vi "Shooter_Sucker_Feed_Mix.vi"(2 "Axis_Y":dbl, 3 "Axis_X":dbl) -> (0 "Suck_Feeder_Out":dbl, 1 "Shoot_Feeder_Out":dbl)   [LabVIEW 2011]
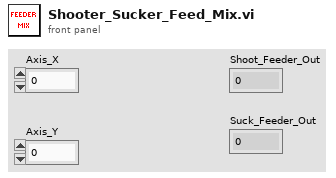
[diagram p1: front panel]
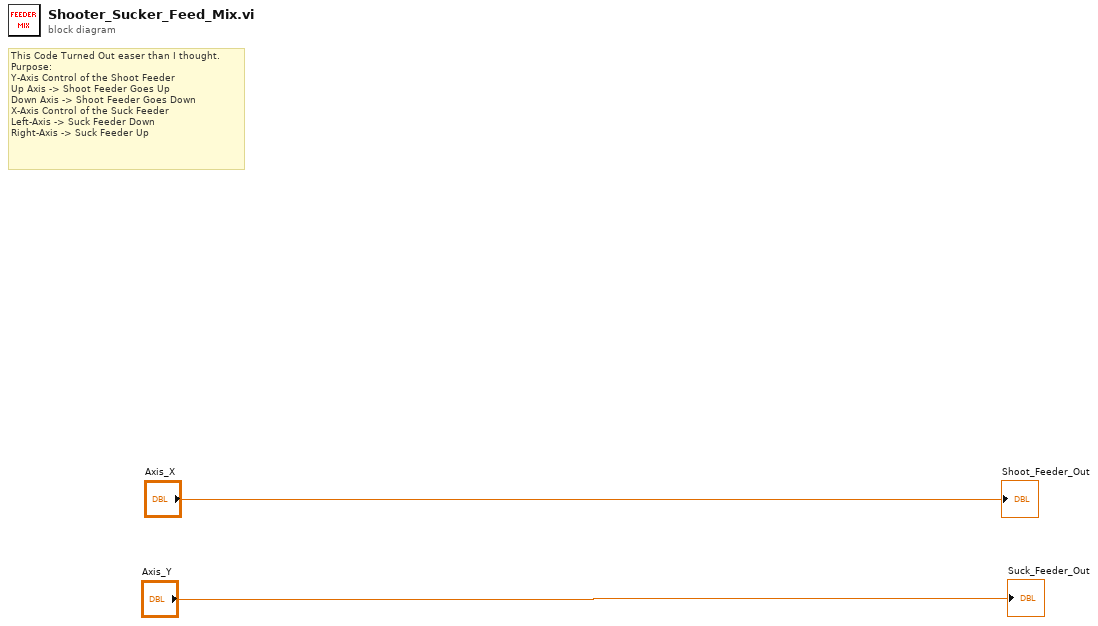
[diagram p0: block diagram]
diagram:
  # "This Code Turned Out easer than I thought. \nPurpose:\nY-Axis Control of the Shoot Feeder\nUp Axis -> Shoot Feeder Goes Up\nDown Axis -> Shoot Feeder Goes Down\nX-Axis Control of the Suck Feeder\nLeft-Axis -> Suck Feeder Down\nRight-Axis -> Suck Feeder Up"
  "Suck_Feeder_Out" <- "Axis_Y"
  "Shoot_Feeder_Out" <- "Axis_X"
